vi "S2DS_Add project.vi"(8 "error in (no error)":errorcluster, 9 "Your name":string, 10 "Add new project":string) -> (0 "error out":errorcluster)   [LabVIEW 2025]
uses:
  <vilib>/Utility/config.llb/Read Key (I32).vi
  <vilib>/Utility/config.llb/Write Key (I32).vi
  <vilib>/Utility/config.llb/Write Key (String).vi
  <vilib>/Utility/config.llb/NI_LVConfig.lvlib
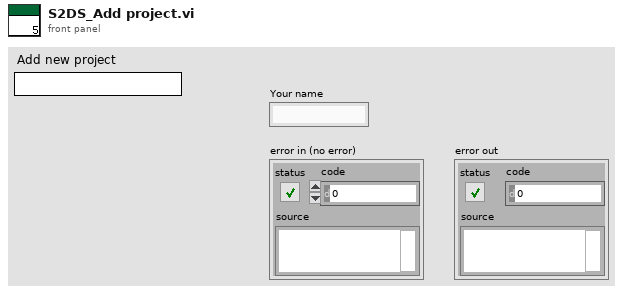
[diagram p1: front panel]
types:
  T1 = typedef "NI_LVConfig.lvlib/Config Data RefNum.ctl" = refnum<k1>
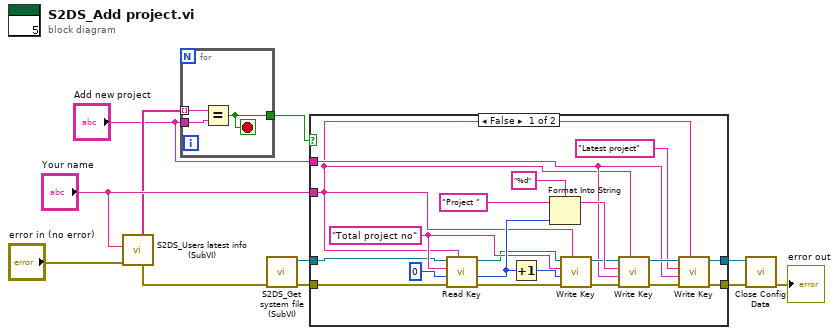
[diagram p0: block diagram]
diagram:
  n1 = call "S2DS_Users latest info (SubVI).vi"("error in (no error)"="error in (no error)", "User name"="Your name") -> ("error out"=w2:errorcluster, "Project list"=w5:string[])  [unwired: 3 in, 5 out]
  n2 = for {
    tunnel: w5 -> [w13] mode=indexing
    tunnel: "Add new project" -> [w14]
    tunnel: [w12] -> w1
    stop <- w12 stop-if-true
    n3 = Equal?(x=w13, y=w14) -> (x = y?=w12:bool)
  }
  n4 = call "S2DS_Get system file (SubVI).vi"("error in (no error)"=w2) -> ("error out"=w11:errorcluster, "Refnum out"=w10:T1)  [unwired: 9 in]
  n5 = case shown="False" w1 {
    tunnel: [w34 w35] -> w8
    tunnel: [w33 w36] -> w9
    tunnel: w11 -> [w18 w35]
    tunnel: w10 -> [w17 w36]
    tunnel: "Add new project" -> [w16 _]
    tunnel: "Your name" -> [w15 _]
    frame False {
      w22 = "Total project no" ("key")
      n6 = call-poly <vilib>:"Read Key.vi"("section"=w15, "error in (no error)"=w18, "default value"=0, "key"=w22, "refnum"=w17) -> ("error out"=w20:errorcluster, "value"=w28:i32, "refnum out"=w19:T1)  [unwired: 3 in, 1 out]
      n7 = Increment(x=w28) -> (x+1=w21:i32)
      n8 = Format Into String(format string="%d", initial string="Project ", w28) -> (resulting string=w29:string)  [unwired: 1 in, 1 out]
      n9 = call-poly <vilib>:"Write Key.vi"("section"=w15, "error in (no error)"=w20, "value"=w21, "key"=w22, "refnum"=w19) -> ("error out"=w24:errorcluster, "refnum out"=w23:T1)  [unwired: 4 in, 1 out]
      n10 = call-poly <vilib>:"Write Key.vi"("section"=w15, "error in (no error)"=w24, "value"=w16, "key"=w29, "refnum"=w23) -> ("error out"=w32:errorcluster, "refnum out"=w31:T1)  [unwired: 4 in, 1 out]
      n11 = call-poly <vilib>:"Write Key.vi"("section"=w15, "error in (no error)"=w32, "value"=w16, "key"="Latest project", "refnum"=w31) -> ("error out"=w34:errorcluster, "refnum out"=w33:T1)  [unwired: 4 in, 1 out]
    }
    frame True {
    }
  }
  n12 = call <vilib>:"Close Config Data.vi"("error in (no error)"=w8, "refnum"=w9) -> ("error out"=→"error out":errorcluster)  [unwired: 8 in, 1 out]
